vi "Write TCP Ref.vi"(8 "error in (no error)":errorcluster, 10 "TCP Ref":refnum<k5>, 11 "Ethernet in":refnum<class "TCP.lvclass">) -> (0 "error out":errorcluster, 3 "Ethernet out":refnum<class "TCP.lvclass">)   [LabVIEW 2019, in "Localhost Protocols.lvlib" / "TCP.lvclass"]
uses:
  TCP.lvclass
  TCP.lvclass/TCP.ctl
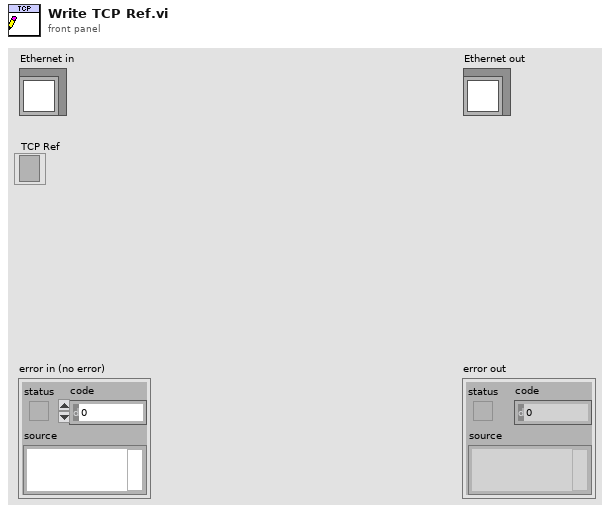
[diagram p1: front panel]
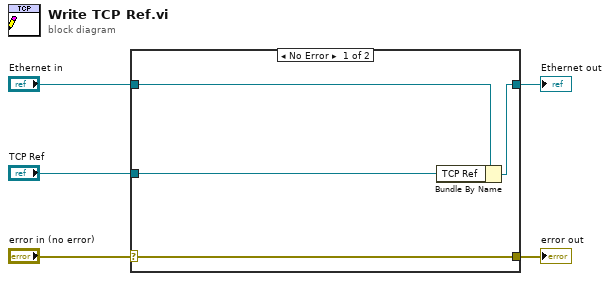
[diagram p0: block diagram]
diagram:
  n1 = case shown="No Error" "error in (no error)" {
    selector: "error in (no error)" -> [w9 w10]
    tunnel: [w9 w10] -> w4
    tunnel: [w7 w11] -> w2
    tunnel: "Ethernet in" -> [w8 w11]
    tunnel: "TCP Ref" -> [w6 _]
    frame No Error {
      n2 = Bundle By Name(cluster=w8, "TCP Ref"=w6) -> (w7:refnum<class "TCP.lvclass">)
    }
    frame Error {
    }
  }
  "error out" <- w4
  "Ethernet out" <- w2
